vi "Graph Update.vi"(7 "Graph Type":enum16{"Combined", "Multiple"}(ring), 10 "Graph Plots":T1(array[cluster]), 11 "Graph Reference in":refnum<vi>[](array[refnum])) -> (3 "Graph Reference out":refnum<vi>[](array[refnum]))   [LabVIEW 2023]
doc: "Use this VI to feed in plot(s) to graph(s). \n\nCombine: Multiple Plots in a single graph.\nSeparated: Single Plot in a graph."
panel:
  out "error out":errorcluster
  in  "error in":errorcluster
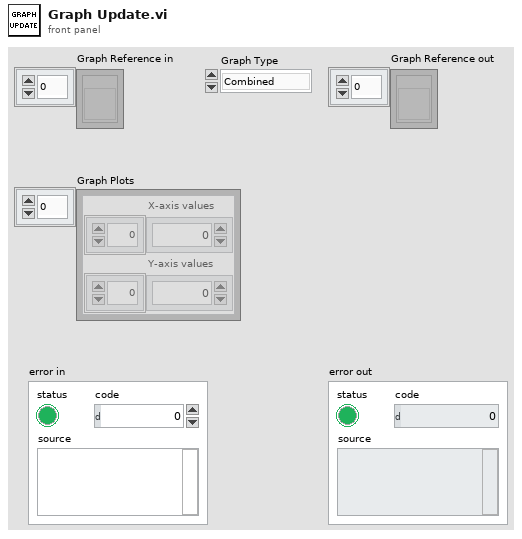
[diagram p1: front panel]
types:
  T1 = cluster{"X-axis values":dbl[], "Y-axis values":dbl[]}[]
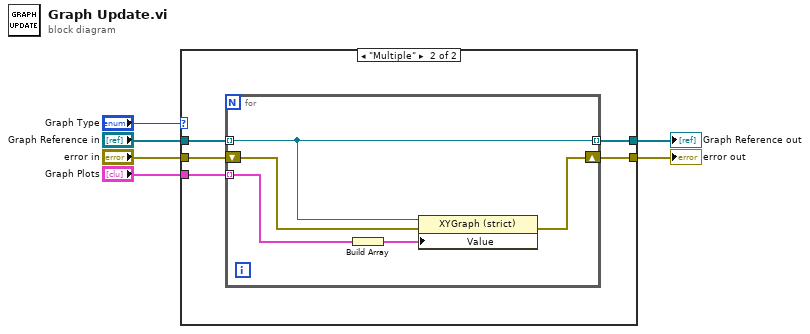
[diagram p0: block diagram]
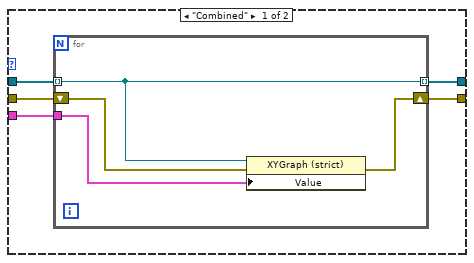
[diagram p2: hidden frame]
diagram:
  n1 = case shown="\"Multiple\"" "Graph Type" {
    tunnel: "Graph Plots" -> [w11 w20]
    tunnel: [w10 w19] -> w1
    tunnel: "error in" -> [w9 w18]
    tunnel: "Graph Reference in" -> [w8 w17]
    tunnel: [w7 w16] -> w3
    frame "Combined" {
      n2 = for {
        tunnel: w11 -> [w15]
        tunnel: w8 -> [w12] mode=indexing
        shift-right: [w14] -> w10
        shift-left: w9 -> [w13]
        tunnel: [w12] -> w7 mode=indexing
        n3 = property on="Property Node" class="XYGraph (strict)"(reference=w12, error in=w13, "Value"=w15) -> (error out=w14:errorcluster)  [unwired: 1 out]
      }
    }
    frame "Multiple" {
      n4 = for {
        tunnel: w20 -> [w25] mode=indexing
        tunnel: w17 -> [w21] mode=indexing
        shift-right: [w24] -> w19
        shift-left: w18 -> [w23]
        tunnel: [w21] -> w16 mode=indexing
        n5 = Build Array(w25) -> (w22:T1)
        n6 = property on="Property Node" class="XYGraph (strict)"(reference=w21, error in=w23, "Value"=w22) -> (error out=w24:errorcluster)  [unwired: 1 out]
      }
    }
  }
  "Graph Reference out" <- w3
  "error out" <- w1
